vi "_Measure Transfer Function_mod1.vi"() -> ()   [LabVIEW 2014]
uses:
  <vilib>/Analysis/4window.llb/windowTd.ctl
  <vilib>/Analysis/1siggen.llb/Ramp Pattern by Samples.vi
  <vilib>/measure/maspectr.llb/FFT Power Spectrum and PSD for 1 Chan.vi
  <vilib>/measure/maspectr.llb/Frequency Response Function (Mag-Phase) 1-1.vi
  <vilib>/Analysis/NI_AALBase.lvlib
  <vilib>/measure/NI_MAPro.lvlib
  <vilib>/Analysis/NI_AALPro.lvlib
panel:
  out "tmr 2 rld value":u16
  out "Phase response":cluster{dbl[], dbl[]}(graph)
  out "Magnitude response":cluster{dbl[], dbl[]}(graph)
  in  "Sweep points":i32=30
  in  "Sweep end [Hz]":dbl=1000.0
  in  "Sweep start [Hz]":dbl=1.0
  in  "Elemszam":u8
  out "VISA Refnum out":refnum<visa-resource-name>
  out "error out":errorcluster
  in  "VISA Refnum in":refnum<visa-resource-name>
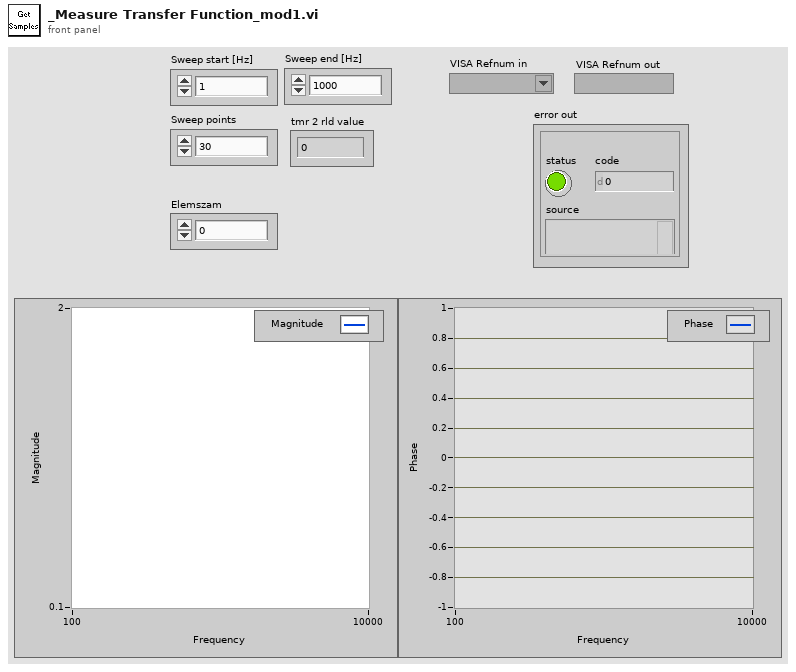
[diagram p1: front panel]
types:
  T1 = typedef "NI_AALPro.lvlib/windowTd.ctl" = u32
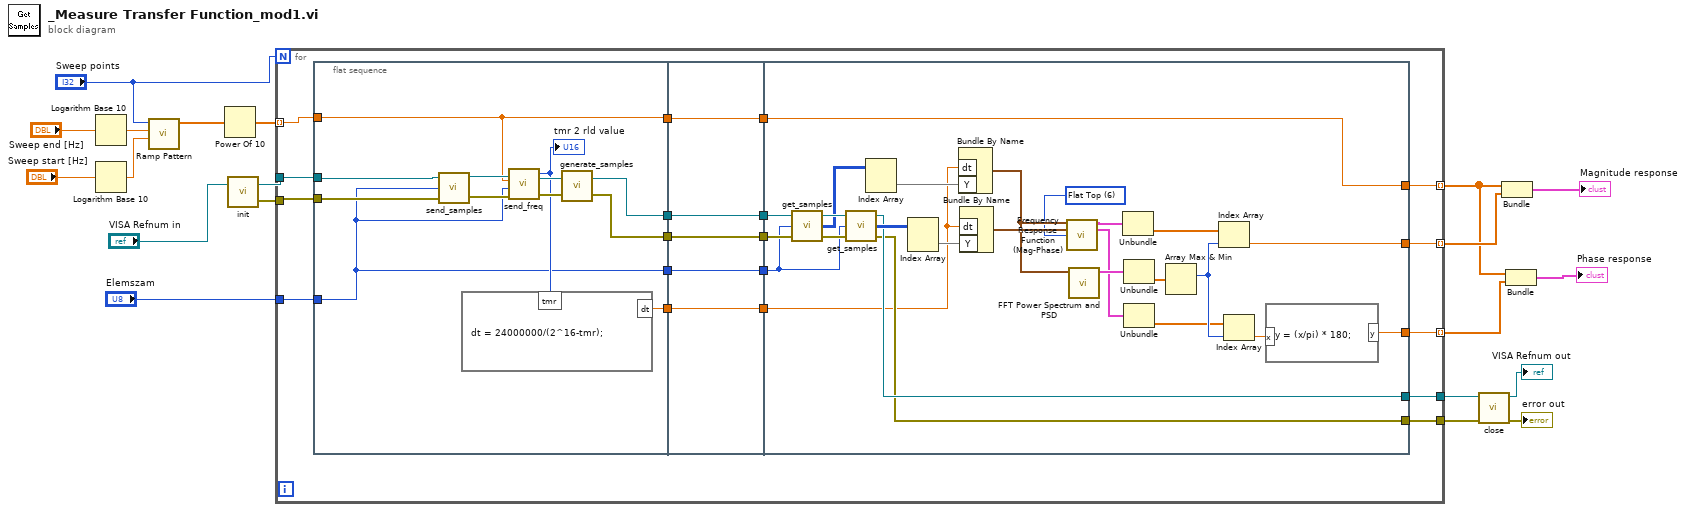
[diagram p0: block diagram]
diagram:
  n1 = Logarithm Base 10(1:"Sweep end [Hz]") -> (0:w19:dbl)
  n2 = Logarithm Base 10(1:"Sweep start [Hz]") -> (0:w17:dbl)
  n3 = call-poly <vilib>:"Ramp Pattern.vi"("start"=w17, "end"=w19, "samples"="Sweep points") -> ("Ramp Pattern"=w20:dbl[])  [unwired: 7 in, 1 out]
  n4 = Power Of 10(x=w20) -> (10^x=w12:dbl[])
  n5 = call "init.vi"("VISA Refnum in"="VISA Refnum in") -> ("error out"=w13:errorcluster, "VISA Refnum out"=w14:refnum<visa-resource-name>)  [unwired: 1 in]
  n6 = for {
    N: "Sweep points" -> [_]
    tunnel: w14 -> [w35]
    tunnel: w13 -> [w34]
    tunnel: w12 -> [w32] mode=indexing
    tunnel: "Elemszam" -> [w33]
    tunnel: [w39] -> w7
    tunnel: [w38] -> w6
    tunnel: [w37] -> w5 mode=indexing
    tunnel: [w36] -> w4 mode=indexing
    tunnel: [w21] -> w1 mode=indexing
    n7 = flat-sequence {
      tunnel: w35 -> [w46]
      tunnel: w34 -> [w45]
      tunnel: w33 -> [w41]
      tunnel: w32 -> [w40]
      tunnel: [w44] -> w30
      tunnel: [w43] -> w29
      tunnel: [w42] -> w26
      tunnel: [w41] -> w25
      tunnel: [w40] -> w23
      tunnel: [w56] -> w31
      tunnel: w30 -> [w56]
      tunnel: w29 -> [w55]
      tunnel: [w55] -> w28
      tunnel: [w54] -> w27
      tunnel: w26 -> [w54]
      tunnel: w25 -> [w53]
      tunnel: [w53] -> w24
      tunnel: w23 -> [w52]
      tunnel: [w52] -> w22
      tunnel: [w65] -> w39
      tunnel: [w64] -> w38
      tunnel: [w63] -> w37
      tunnel: [w62] -> w36
      tunnel: w31 -> [w61]
      tunnel: w28 -> [w60]
      tunnel: w27 -> [w59]
      tunnel: w24 -> [w58]
      tunnel: w22 -> [w57]
      tunnel: [w57] -> w21
      frame #0 {
        n8 = call "send_samples.vi"("error in (no error)"=w45, "elemszam"=w41, "VISA Refnum in"=w46) -> ("error out"=w51:errorcluster, "VISA Refnum out"=w50:refnum<visa-resource-name>)
        n9 = call "send_freq.vi"("error in (no error)"=w51, "elemszam"=w41, "signal freq"=w40, "VISA Refnum in"=w50) -> ("error out"=w48:errorcluster, "VISA Refnum out"=w49:refnum<visa-resource-name>, "tmr 2 rld value"=w47:u16)
        "tmr 2 rld value" <- w47
        n10 = formula code="dt = 24000000/(2^16-tmr);"("tmr"=w47) -> ("dt"=w42:dbl)
        n11 = call "generate_samples.vi"("error in (no error)"=w48, "VISA Refnum in"=w49) -> ("error out"=w43:errorcluster, "VISA Refnum out"=w44:refnum<visa-resource-name>)
      }
      frame #1 {
      }
      frame #2 {
        w70 = T1 6 items=["Rectangle"=0, "Hanning"=1, "Hamming"=2, "Blackman-Harris"=3, "Exact Blackman"=4, "Blackman"=5, "Flat Top"=6, "4 Term B-Harris "=7, "7 Term B-Harris"=8, "Low Sidelobe"=9, "Blackman Nuttall"=11, "Triangle"=30, "Bartlett-Hanning"=31, "Bohman"=32, "Parzen"=33, "Welch"=34, "Kaiser"=60, "Dolph-Chebyshev"=61, "Gaussian"=62] ("window")
        n12 = call "get_samples.vi"("error in (no error)"=w60, "#Samples to read"=w58, "VISA Refnum in"=w61) -> ("error out"=w82:errorcluster, "Array"=w66:u16[][], "VISA Refnum out"=w81:refnum<visa-resource-name>)
        n13 = call "get_samples.vi"("error in (no error)"=w82, "#Samples to read"=w58, "VISA Refnum in"=w81) -> ("error out"=w64:errorcluster, "Array"=w78:u16[][], "VISA Refnum out"=w65:refnum<visa-resource-name>)
        n14 = Index Array(array=w66) -> (element=w79:u16[])  [unwired: 2 in]
        n15 = Index Array(array=w78) -> (element=w80:u16[])  [unwired: 2 in]
        n16 = Bundle By Name("dt"=w59, "Y"=w79) -> (w75:waveform(u16))  [unwired: 1 in]
        n17 = Bundle By Name("dt"=w59, "Y"=w80) -> (w76:waveform(u16))  [unwired: 1 in]
        n18 = call-poly <vilib>:"Frequency Response Function (Mag-Phase).vi"("time signal X"=w75, "time signal Y"=w76, "window"=w70) -> ("magnitude"=w72:cluster{"f0":dbl, "df":dbl, "magnitude":dbl[]}, "phase"=w69:cluster{"f0":dbl, "df":dbl, "phase":dbl[]})  [unwired: 7 in, 4 out]
        n19 = call-poly <vilib>:"FFT Power Spectrum and PSD.vi"("time signal"=w75) -> ("Power Spectrum / PSD"=w71:cluster{"f0":dbl, "df":dbl, "magnitude":dbl[]})  [unwired: 7 in, 3 out]
        n20 = Unbundle(w72) -> ("magnitude"=w73:dbl[])  [unwired: 2 out]
        n21 = Unbundle(w71) -> ("magnitude"=w67:dbl[])  [unwired: 2 out]
        n22 = Unbundle(w69) -> ("phase"=w68:dbl[])  [unwired: 2 out]
        n23 = Array Max & Min(array=w67) -> (max index (indices)=w74:i32)  [unwired: 3 out]
        n24 = Index Array(array=w73, index=w74) -> (element=w63:dbl)
        n25 = Index Array(array=w68, index=w74) -> (element=w77:dbl)
        n26 = formula code="y = (x/pi) * 180;"("x"=w77) -> ("y"=w62:dbl)
      }
    }
  }
  n27 = call "close.vi"("error in (no error)"=w6, "VISA resource name"=w7) -> ("error out"=→"error out":errorcluster, "VISA resource name out"=→"VISA Refnum out":refnum<visa-resource-name>)  [unwired: 4 in]
  n28 = Bundle(w1, w5) -> (→"Magnitude response":cluster{dbl[], dbl[]})  [unwired: 1 in]
  n29 = Bundle(w1, w4) -> (→"Phase response":cluster{dbl[], dbl[]})  [unwired: 1 in]
